vi "To TYPE Line.vi"(8 "error in (no error)":errorcluster, 10 "Name":string, 11 "Metric":refnum<data-value>) -> (0 "error out":errorcluster, 3 "TYPE line":string)   [LabVIEW 2020, in "Metrics.lvlib" / "Metric.lvclass"]
uses:
  Metric.lvclass
  <vilib>/regexp/Match Regular Expression.xnode
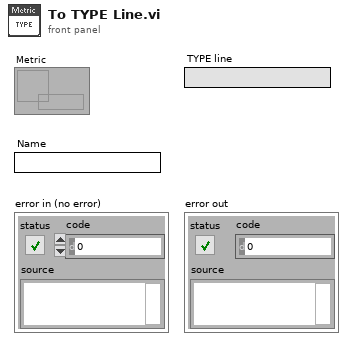
[diagram p1: front panel]
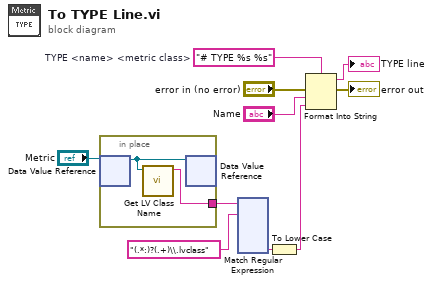
[diagram p0: block diagram]
diagram:
  w5 = "# TYPE %s %s"  # TYPE <name> <metric class>
  n1 = in-place {
    in-place-border: [w12] -> w3
    n2 = in-place-dvr #1("Metric") -> (w11:refnum<class "Metric.lvclass">)  [unwired: 1 out]
    n3 = call <vilib>:"Get LV Class Name.vi"("object"=w11) -> ("class name"=w12:string)  [unwired: 9 in, 1 out]
    n4 = in-place-dvr #1(w11) -> ()  [unwired: 2 out]
  }
  n5 = xnode "Match Regular Expression"("input string"=w3, "regular expression"="(.*:)?(.+)\\.lvclass") -> ("submatch 2"=w8:string)  [unwired: 4 in, 6 out]
  n6 = To Lower Case(string=w8) -> (all lower case string=w1:string)
  n7 = Format Into String(format string=w5, error in="error in (no error)", "Name", w1) -> (resulting string=→"TYPE line":string, error out=→"error out":errorcluster)  [unwired: 1 in]
